vi "MAX-MeasureVoltage_DAQAssistant_SixChannels_V2.vi"() -> ()   [LabVIEW 2017]
panel:
  out "data":dynamicdata(graph)
  out "SF3":dbl
  out "SF2":dbl
  out "SF1":dbl
  out "D1":dbl
  out "L2":dbl
  out "L1":dbl
  in  "file path":path=path "D:/Users/UWAIARG2/Documents/test4.tdms"
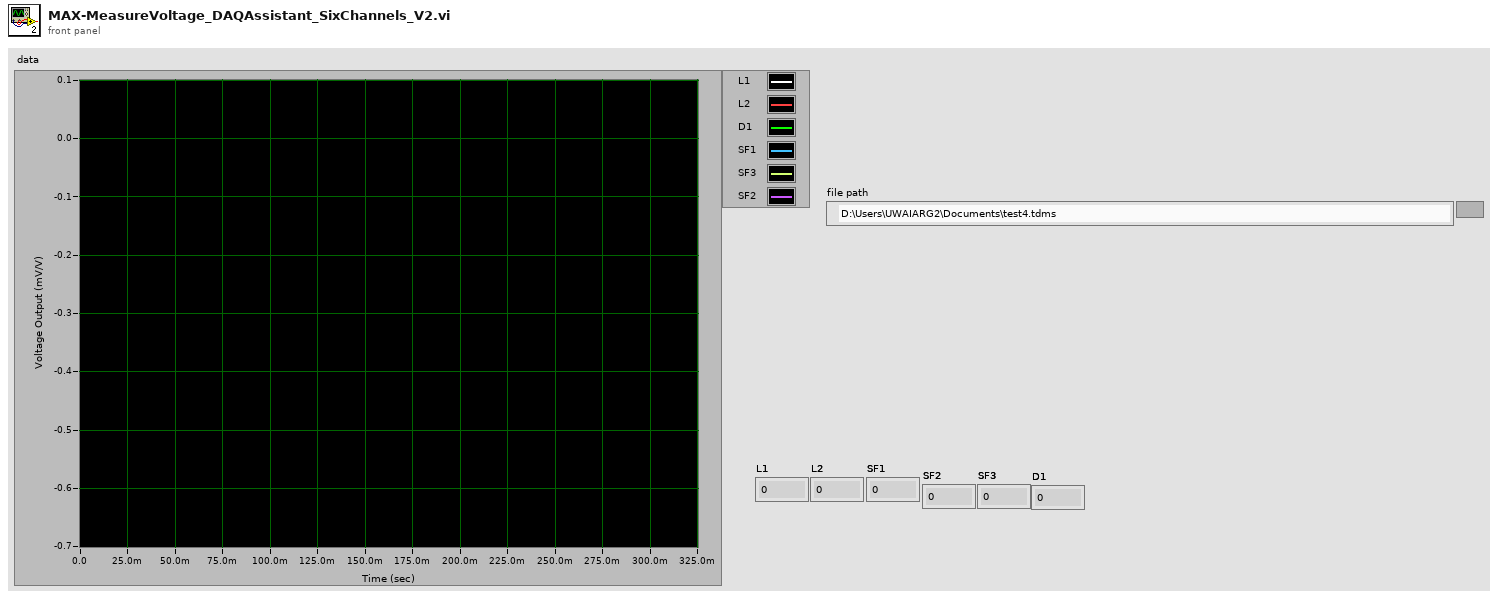
[diagram p1: front panel]
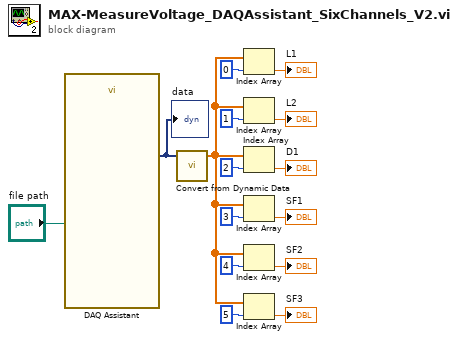
[diagram p0: block diagram]
diagram:
  n1 = call "DAQ Assistant"("file path"="file path") -> ("data"=w14:dynamicdata)  [unwired: 16 in, 2 out]
  "data" <- w14
  n2 = call "Convert from Dynamic Data"("Dynamic Data Type"=w14) -> ("Array"=w5:dbl[])  [unwired: 3 in]
  n3 = Index Array(array=w5, index=0) -> (element=→"L1":dbl)
  n4 = Index Array(array=w5, index=1) -> (element=→"L2":dbl)
  n5 = Index Array(array=w5, index=2) -> (element=→"D1":dbl)
  n6 = Index Array(array=w5, index=3) -> (element=→"SF1":dbl)
  n7 = Index Array(array=w5, index=4) -> (element=→"SF2":dbl)
  n8 = Index Array(array=w5, index=5) -> (element=→"SF3":dbl)
